vi "Close.vi"(8 "error in (no error)":errorcluster, 10 "Write if modified? (T)":bool=TRUE, 11 "LabVIEW-Config.lvlib:LabVIEW-Config.lvclass":refnum<class "LabVIEW-Config.lvclass">) -> (0 "error out":errorcluster, 3 "Path":path)   [LabVIEW 2017, in "LabVIEW-Config.lvlib" / "LabVIEW-Config.lvclass"]
uses:
  LabVIEW-Config.lvclass
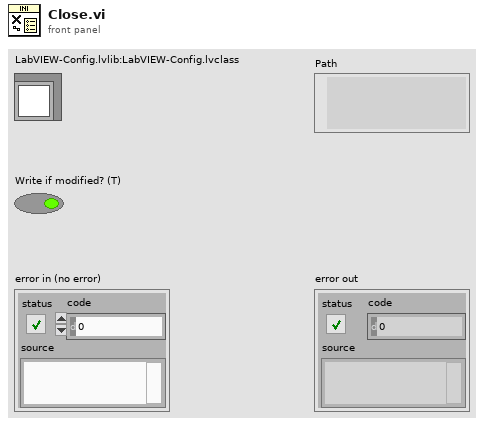
[diagram p1: front panel]
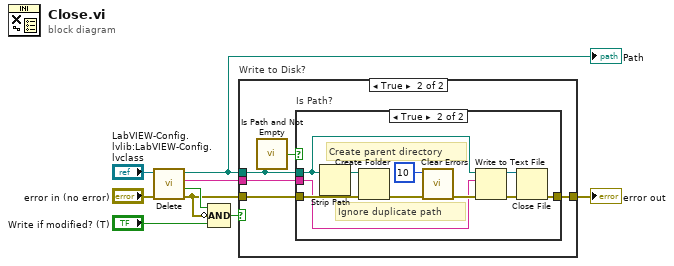
[diagram p0: block diagram]
diagram:
  n1 = call "Delete.vi"("error in (no error)"="error in (no error)", "LabVIEW-Config.lvlib:LabVIEW-Config.lvclass"="LabVIEW-Config.lvlib:LabVIEW-Config.lvclass") -> ("error out"=w1:errorcluster, "Modified?"=w3:bool, "Text"=w2:string, "Path"=w4:path)  [unwired: 6 in]
  "Path" <- w4
  n2 = Compound Arithmetic op=AND(w3, invert w1, "Write if modified? (T)") -> (w7:bool)
  n3 = case "Write to Disk?" shown="True" w7 {
    tunnel: w1 -> [w10 w12]
    tunnel: [w10 w15] -> w8
    tunnel: w4 -> [_ w14]
    tunnel: w2 -> [_ w13]
    frame False {
    }
    frame True {
      n4 = call <vilib>:"Is Path and Not Empty.vi"("path"=w14) -> ("Is Path and Not Empty?"=w11:bool)  [unwired: 4 in]
      n5 = case "Is Path?" shown="True" w11 {
        tunnel: [w16 w20] -> w15
        tunnel: w14 -> [_ w19]
        tunnel: w13 -> [_ w17]
        tunnel: w12 -> [w16 w18]
        frame False {
        }
        frame True {
          # "Create parent directory"
          # "Ignore duplicate path"
          n6 = Strip Path(path=w19) -> (stripped path=w25:path)  [unwired: 1 out]
          n7 = Create Folder(path (use dialog)=w25, error in=w18) -> (error out=w23:errorcluster)  [unwired: 1 in, 2 out]
          n8 = call <vilib>:"Clear Errors.vi"("error in (no error)"=w23, "specific error code to clear (0: all)"=10 ("Not Found")) -> ("error out"=w26:errorcluster)  [unwired: 4 in, 1 out]
          n9 = Write to Text File(file (use dialog)=w19, text=w17, error in=w26) -> (refnum out=w21:refnum<file>, error out=w22:errorcluster)  [unwired: 1 in, 1 out]
          n10 = Close File(refnum=w21, error in=w22) -> (error out=w20:errorcluster)  [unwired: 1 out]
        }
      }
    }
  }
  "error out" <- w8
